vi "hexStringLength.vi"(1 "byte order (little-endian)":T1(ring)=enum."little-endian", 2 "byte length (4)":i32=4 min=1 max=4, 3 "String":string) -> (0 "String hex length":string)   [LabVIEW 2012]
panel:
  out "String Length":i32
  # "Gives Length as Little Endian"
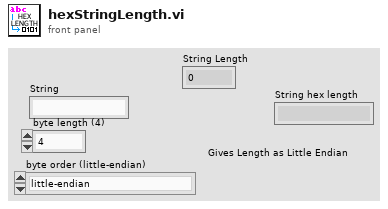
[diagram p1: front panel]
types:
  T1 = enum16{"big-endian, network order", "native, host order", "little-endian"}
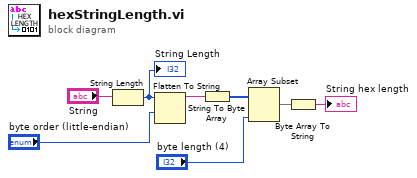
[diagram p0: block diagram]
diagram:
  n1 = String Length(string="String") -> (length=w6:i32)
  "String Length" <- w6
  n2 = Flatten To String(anything=w6, byte order (0:big-endian, network order)="byte order (little-endian)") -> (data string=w5:string)  [unwired: 2 in, 2 out]
  n3 = String To Byte Array(string=w5) -> (unsigned byte array=w4:u8[])
  n4 = Array Subset(array=w4, length="byte length (4)") -> (w3:u8[])  [unwired: 1 in]
  n5 = Byte Array To String(unsigned byte array=w3) -> (string=→"String hex length":string)
